vi "example_asynch_wait_2.vi"() -> ()   [LabVIEW 2015]
uses:
  polys/poly_asynch_wait_wait.vi
  cores/core_timing_tools_eco.vi
  polys/poly_timing_tools_eco_plus.vi
  ref_tools/name_of_caller.vi
  cast_boolean_notifier.vi
  polys/poly_cast_boolean_notifier_n2q.vi
  polys/poly_cast_boolean_notifier_q2n.vi
  polys/poly_asynch_wait_start.vi
  loop_timeout.vi
  polys/poly_loop_timeout_bool.vi
  error_tools/merge_errors.vi
  error_tools/polys/poly_merge_errors_down.vi
  error_tools/toolbox_error_handler.vi
  <vilib>/Utility/error.llb/Simple Error Handler.vi
  polys/poly_asynch_wait_stop.vi
  polys/poly_asynch_wait_notify.vi
panel:
  out "name":string
  out "notifications":i32 format="- %.0f -"
  in  "notify":bool
  out "timeouts":i32 format="- %.0f -"
  in  "timeout":i32=300 format="%.0f ms"
  in  "stop":bool
  # "notifier name"
  # "timeout [ms]"
  # "timeouts"
  # "notif.s"
  # "send notif."
  # "stop"
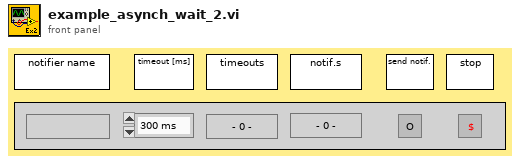
[diagram p1: front panel]
types:
  T1 = typedef "boolean_notifier.ctl" = refnum<k1>
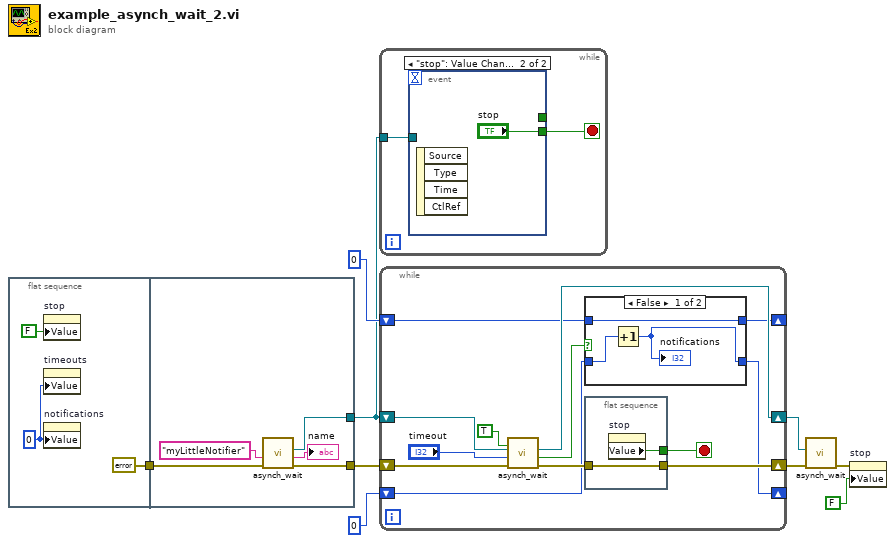
[diagram p0: block diagram]
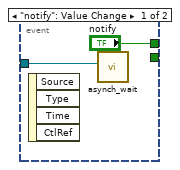
[diagram p2: hidden frame]
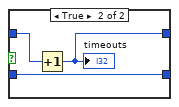
[diagram p3: hidden frame]
diagram:
  n1 = flat-sequence {
    tunnel: [errorcluster {"status"=FALSE, "code"=0, "source"=""} ("error constant")] -> w5
    tunnel: w5 -> [w15]
    tunnel: [w17] -> w4
    tunnel: [w14] -> w3
    frame #0 {
      w11 = 0
      n2 = property on="stop" class="Bool (strict)"("Value"=FALSE) -> ()  [unwired: 2 in, 2 out]
      n3 = property on="timeouts" class="DigNum (strict)"("Value"=w11) -> ()  [unwired: 2 in, 2 out]
      n4 = property on="notifications" class="DigNum (strict)"("Value"=w11) -> ()  [unwired: 2 in, 2 out]
    }
    frame #1 {
      n5 = call-poly "asynch_wait.vi"("error in"=w15, "notifier name"="myLittleNotifier") -> ("error out"=w14:errorcluster, "notifier name"=→"name":string, "notifier"=w17:T1)  [unwired: 7 in]
    }
  }
  n6 = while {
    tunnel: w4 -> [w19]
    stop <- w18 stop-if-true
    n7 = event shown="[1] \"stop\": Value Change" {
      selector: _ -> [_ _]
      dyn-events: _ -> [_ _]
      timeout: _ -> [_ _]
      tunnel: w19 -> [w21 _]
      tunnel: ["notify" _] -> _
      tunnel: [_ "stop"] -> w18
      event "notify": Value Change {
        n8 = event-data() -> ()  [unwired: 1 in, 4 out]
        n9 = call-poly "asynch_wait.vi"("notifier"=w21) -> ()  [unwired: 9 in, 2 out]
      }
      event "stop": Value Change {
        n10 = event-data() -> ()  [unwired: 1 in, 4 out]
      }
    }
  }
  n11 = while {
    shift-right: [w31] -> w9
    shift-left: w4 -> [w32]
    shift-right: [w29] -> w8
    shift-left: w3 -> [w34]
    shift-right: [w25] -> _
    shift-left: 0 -> [w26]
    shift-right: [w23] -> _
    shift-left: 0 -> [w24]
    stop <- w28 stop-if-true
    n12 = call-poly "asynch_wait.vi"("keep waiting? (F)"=TRUE, "error in"=w34, "timeout"="timeout", "notifier"=w32) -> ("error out"=w30:errorcluster, "timed out?"=w27:bool, "notifier out"=w31:T1)  [unwired: 5 in]
    n13 = case shown="False" w27 {
      tunnel: w26 -> [w38 w41]
      tunnel: [w38 w39] -> w25
      tunnel: w24 -> [w37 w40]
      tunnel: [w36 w40] -> w23
      frame False {
        n14 = Increment(x=w37) -> (x+1=w36:i32)
        "notifications" <- w36
      }
      frame True {
        n15 = Increment(x=w41) -> (x+1=w39:i32)
        "timeouts" <- w39
      }
    }
    n16 = flat-sequence {
      tunnel: [w42] -> w28
      tunnel: [w43] -> w29
      tunnel: w30 -> [w43]
      frame #0 {
        n17 = property on="stop" class="Bool (strict)"() -> ("Value"=w42:bool)  [unwired: 2 in, 2 out]
      }
    }
  }
  n18 = call-poly "asynch_wait.vi"("error in"=w8, "notifier"=w9) -> ("error out"=w1:errorcluster)  [unwired: 9 in]
  n19 = property on="stop" class="Bool (strict)"(error in=w1, "Value"=FALSE) -> ()  [unwired: 1 in, 2 out]
